vi "Rename Digital Pattern.vi"(6 "OldVal":string, 8 "error in (no error)":errorcluster, 9 "NewVal":string, 10 "Page Data in":T1 {"Node Ptr" format="%.0x"}, 11 "State Queue in":string[](array[string])) -> (0 "error out":errorcluster, 1 "name collision?":bool, 2 "Page Data out":T1 {"Node Ptr" format="%.0x"}, 3 "State Queue out":string[](array[string]))   [LabVIEW 2020, in "Engine Simulation Toolkit System Explorer.lvlib"]
uses:
  Engine Simulation Toolkit System Explorer.lvlib
  Digital Patterns Page Data.ctl
  <vilib>/NI VeriStand/Custom Device API/Custom Device Item Ref.ctl
  Digital Pattern.ctl
  Digital Pattern Base.ctl
  Digital Pattern Remove Edge.ctl
  Digital Pattern Add Pulse.ctl
  <vilib>/NI VeriStand/Custom Device API/Custom Device API.lvlib
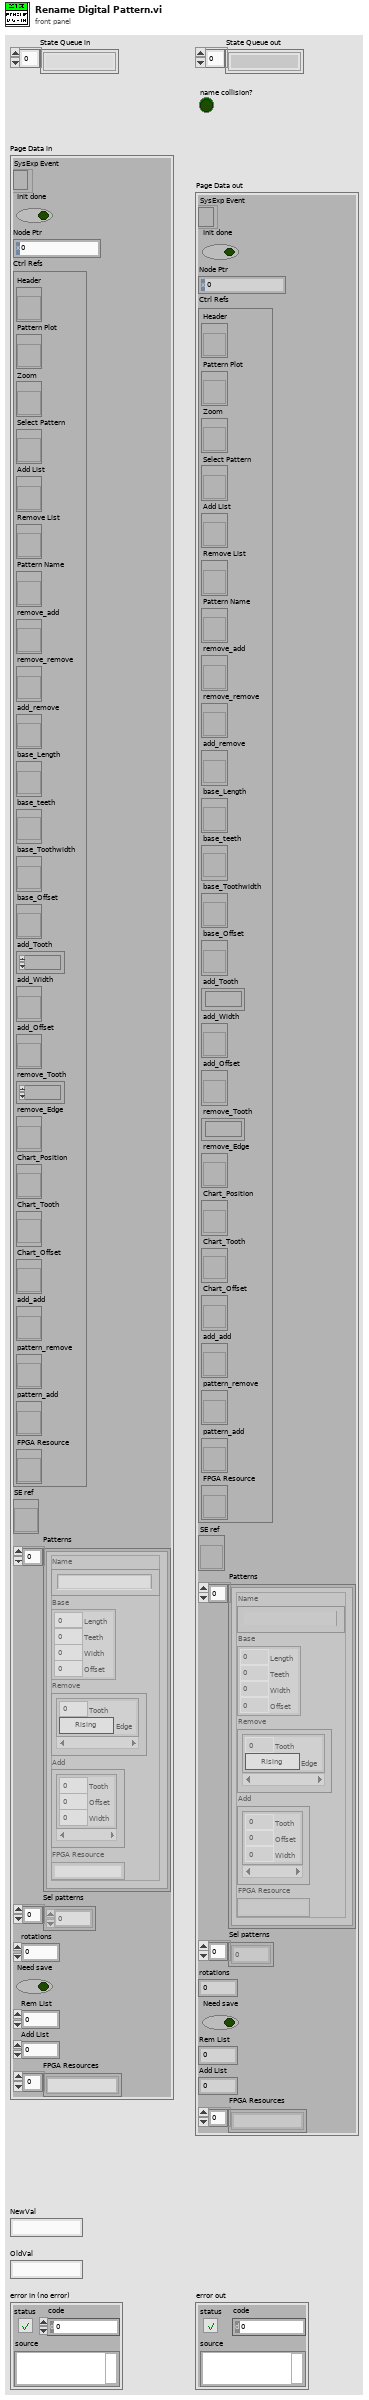
[diagram p1: front panel]
types:
  T1 = typedef "Engine Simulation Toolkit System Explorer.lvlib/Digital Patterns Page Data.ctl" = cluster{"SysExp Event":refnum<event-registration>, "Init done":bool, "Node Ptr":T2, "Ctrl Refs":cluster{"Header":refnum<vi>, "Pattern Plot":refnum<vi>, "Zoom":refnum<vi>, "Select Pattern":refnum<vi>, "Add List":refnum<vi>, "Remove List":refnum<vi>, "Pattern Name":refnum<vi>, "remove_add":refnum<vi>, "remove_remove":refnum<vi>, "add_remove":refnum<vi>, "base_Length":refnum<vi>, "base_teeth":refnum<vi>, "base_Toothwidth":refnum<vi>, "base_Offset":refnum<vi>, "add_Tooth":refnum<vi>, "add_Width":refnum<vi>, "add_Offset":refnum<vi>, "remove_Tooth":refnum<vi>, "remove_Edge":refnum<vi>, "Chart_Position":refnum<vi>, "Chart_Tooth":refnum<vi>, "Chart_Offset":refnum<vi>, "add_add":refnum<vi>, "pattern_remove":refnum<vi>, "pattern_add":refnum<vi>, "FPGA Resource":refnum<vi>}, "SE ref":refnum<vi>, "Patterns":T3[], "Sel patterns":i32[], "rotations":u16, "Need save":bool, "Rem List":i32, "Add List":i32, "FPGA Resources":string[]}
  T2 = typedef "Custom Device API.lvlib/Custom Device Item Ref.ctl" = u64
  T3 = typedef "Engine Simulation Toolkit System Explorer.lvlib/Digital Pattern.ctl" = cluster{"Name":string, "Base":T4, "Remove":T5[], "Add":T6[], "FPGA Resource":string}
  T4 = typedef "Engine Simulation Toolkit System Explorer.lvlib/Digital Pattern Base.ctl" = cluster{"Length":dbl, "Teeth":u16, "Width":dbl, "Offset":dbl}
  T5 = typedef "Engine Simulation Toolkit System Explorer.lvlib/Digital Pattern Remove Edge.ctl" = cluster{"Tooth":u16, "Edge":bool}
  T6 = typedef "Engine Simulation Toolkit System Explorer.lvlib/Digital Pattern Add Pulse.ctl" = cluster{"Tooth":u16, "Offset":dbl, "Width":dbl}
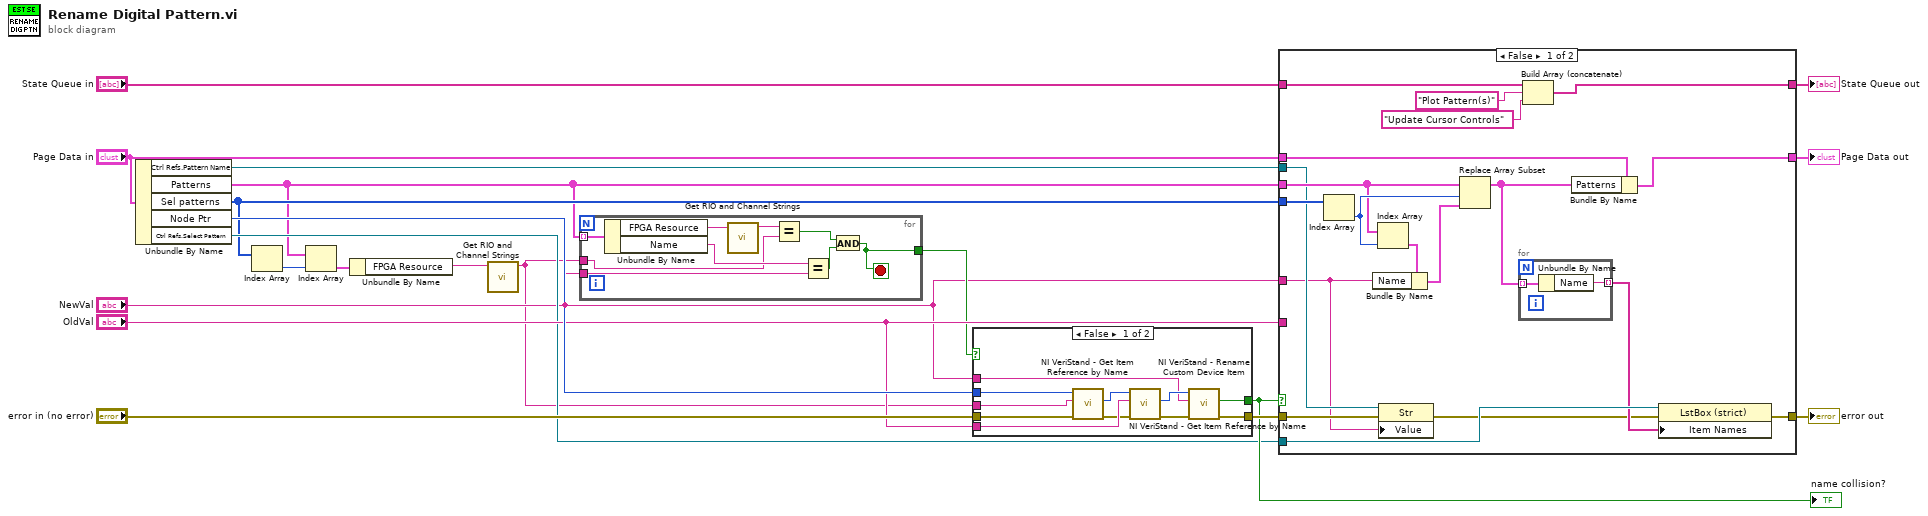
[diagram p0: block diagram]
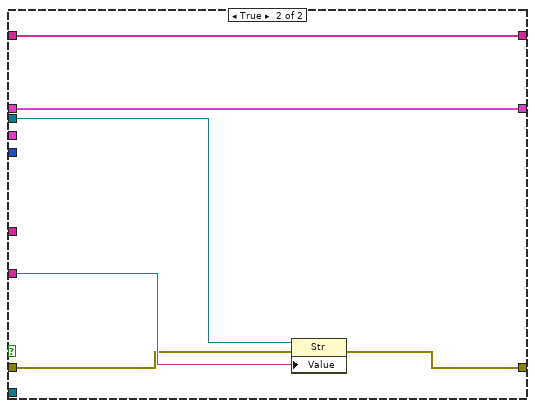
[diagram p3: hidden frame]
diagram:
  n1 = Unbundle By Name("Page Data in") -> ("Ctrl Refs.Pattern Name"=w15:refnum<vi>, "Patterns"=w2:T3[], "Sel patterns"=w8:i32[], "Node Ptr"=w14:T2, "Ctrl Refs.Select Pattern"=w9:refnum<vi>)
  n2 = Index Array(array=w8) -> (element=w7:i32)  [unwired: 1 in]
  n3 = Index Array(array=w2, index=w7) -> (element=w6:T3)
  n4 = Unbundle By Name(w6) -> ("FPGA Resource"=w5:string)
  n5 = call "Get RIO and Channel Strings.vi"("rio/channel"=w5) -> ("rio"=w1:string)  [unwired: 9 in, 1 out]
  n6 = for {
    tunnel: w2 -> [w29] mode=indexing
    tunnel: "NewVal" -> [w21]
    tunnel: [w22] -> w4
    tunnel: w1 -> [w25]
    stop <- w22 stop-if-true
    n7 = Unbundle By Name(w29) -> ("FPGA Resource"=w27:string, "Name"=w28:string)
    n8 = call "Get RIO and Channel Strings.vi"("rio/channel"=w27) -> ("rio"=w26:string)  [unwired: 9 in, 1 out]
    n9 = Equal?(x=w26, y=w25) -> (x = y?=w23:bool)
    n10 = Equal?(x=w28, y=w21) -> (x = y?=w24:bool)
    n11 = And(x=w23, y=w24) -> (x .and. y?=w22:bool)
  }
  n12 = case shown="False" w4 {
    selector: w4 -> [_ w41]
    tunnel: "error in (no error)" -> [w34 w42]
    tunnel: w14 -> [w32 _]
    tunnel: [w38 w42] -> w13
    tunnel: "OldVal" -> [w37 _]
    tunnel: "NewVal" -> [w36 _]
    tunnel: [w35 w41] -> w10
    tunnel: w1 -> [w30 _]
    frame False {
      n13 = call <vilib>:"NI VeriStand - Get Item Reference by Name.vi"("error in (no error)"=w34, "Item Name"=w30, "Parent Ref in"=w32) -> ("error out"=w33:errorcluster, "Item Ref"=w31:T2)  [unwired: 5 in, 2 out]
      n14 = call <vilib>:"NI VeriStand - Get Item Reference by Name.vi"("error in (no error)"=w33, "Item Name"=w37, "Parent Ref in"=w31) -> ("error out"=w39:errorcluster, "Item Ref"=w40:T2)  [unwired: 5 in, 2 out]
      n15 = call <vilib>:"NI VeriStand - Rename Custom Device Item.vi"("error in (no error)"=w39, "New Name"=w36, "Item Ref in"=w40) -> ("error out"=w38:errorcluster, "Request invalid?"=w35:bool)  [unwired: 6 in, 1 out]
    }
    frame True {
    }
  }
  "name collision?" <- w10
  n16 = case shown="False" w10 {
    tunnel: "State Queue in" -> [w61 w68]
    tunnel: w2 -> [w57 _]
    tunnel: w8 -> [w56 _]
    tunnel: "Page Data in" -> [w55 w67]
    tunnel: [w54 w67] -> w18
    tunnel: [w53 w68] -> w19
    tunnel: "OldVal" -> [_ w69]
    tunnel: "NewVal" -> [w43 _]
    tunnel: [w49 w64] -> w20
    tunnel: w13 -> [w46 w65]
    tunnel: w15 -> [w44 w66]
    tunnel: w9 -> [w48 _]
    frame False {
      n17 = Index Array(array=w56) -> (element=w58:i32)  [unwired: 1 in]
      n18 = Index Array(array=w57, index=w58) -> (element=w59:T3)
      n19 = Bundle By Name(cluster=w59, "Name"=w43) -> (w60:T3)
      n20 = property class="Str"(reference=w44, error in=w46, "Value"=w43) -> (error out=w45:errorcluster)  [unwired: 1 out]
      n21 = Replace Array Subset(array=w57, new element=w60, index=w58) -> (w50:T3[])
      n22 = for {
        tunnel: w50 -> [w63] mode=indexing
        tunnel: [w62] -> w47 mode=indexing
        n23 = Unbundle By Name(w63) -> ("Name"=w62:string)
      }
      n24 = Build Array (concatenate)(w61, "Plot Pattern(s)", "Update Cursor Controls") -> (w53:string[])
      n25 = Bundle By Name(cluster=w55, "Patterns"=w50) -> (w54:T1)
      n26 = property class="LstBox (strict)"(reference=w48, error in=w45, "Item Names"=w47) -> (error out=w49:errorcluster)  [unwired: 1 out]
    }
    frame True {
      n27 = property class="Str"(reference=w66, error in=w65, "Value"=w69) -> (error out=w64:errorcluster)  [unwired: 1 out]
    }
  }
  "error out" <- w20
  "State Queue out" <- w19
  "Page Data out" <- w18
